vi "DetermineRegime.vi"(4 "Input Data":T1, 6 "Debug with explicit inputs? (F)":bool, 8 "Last Commanded Boat Regime":T5={"Sailing Regime"=enum."Upwind - Starboard Tack", "Emergency Regimes"=enum."NO EMERGENCY", "Emergency?"=FALSE}, 10 "Desired Heading (deg)":dbl, 11 "NotifierReff":T2) -> (3 "Commanded Boat Regime":T5)   [LabVIEW 2013]
doc: "This VI takes in\n - Trusted absolute wind data (this may be from the wind sensor, or may be frozen from before if the sensor data is bad in a certain area)\n - Robot heading (compass, 0-360)\n - Desired heading (same 0-360)\n - Last commanded regime\n\nThis VI commands a regime, either steady-state or transistion, and tells the Sail and Rudder controller to execute that regime. Documented here: https://docs.google.com/file/d/0B6St7IDGiYunU3FLWTZHTUFHWHc/edit\n\nFeb. 2014, Eric Schneider"
uses:
  Data/TypeDefs/Boat Regimes.ctl
  Data/TypeDefs/Sailing Regimes.ctl
  Data/TypeDefs/Emergency Regimes.ctl
  Data/TypeDefs/Regime Boundaries.ctl
  Data/TypeDefs/Notifiers.ctl
  Data/TypeDefs/UTM Location.ctl
  Data/TypeDefs/Sail Set Suggestions.ctl
  Data/TypeDefs/Rudder Set Suggestions.ctl
  Data/TypeDefs/OverrideInformation.ctl
  Data/TypeDefs/OverrideMode.ctl
  Data/TypeDefs/MotorSetup.ctl
  Data/TypeDefs/DynamixelSetupInfo.ctl
  Data/TypeDefs/AirmarStatus.ctl
panel:
  in  "Allowable Turn Error":dbl=5.0
  out "HasTransitionFailed?":bool
  out "Altered regime boundaries":T3=[0, 70, 140, 220, 190, 360]
  out "ShouldWeChangeRegime?":bool
  out "Desired Steady State Regime":T4
  out "Current Steady-State Regime":T4
  out "Are We In Transition?":bool
  # "These controls are only used for debugging, see the Midbrain Tests folder"
  # "FOR DEBUGGING"
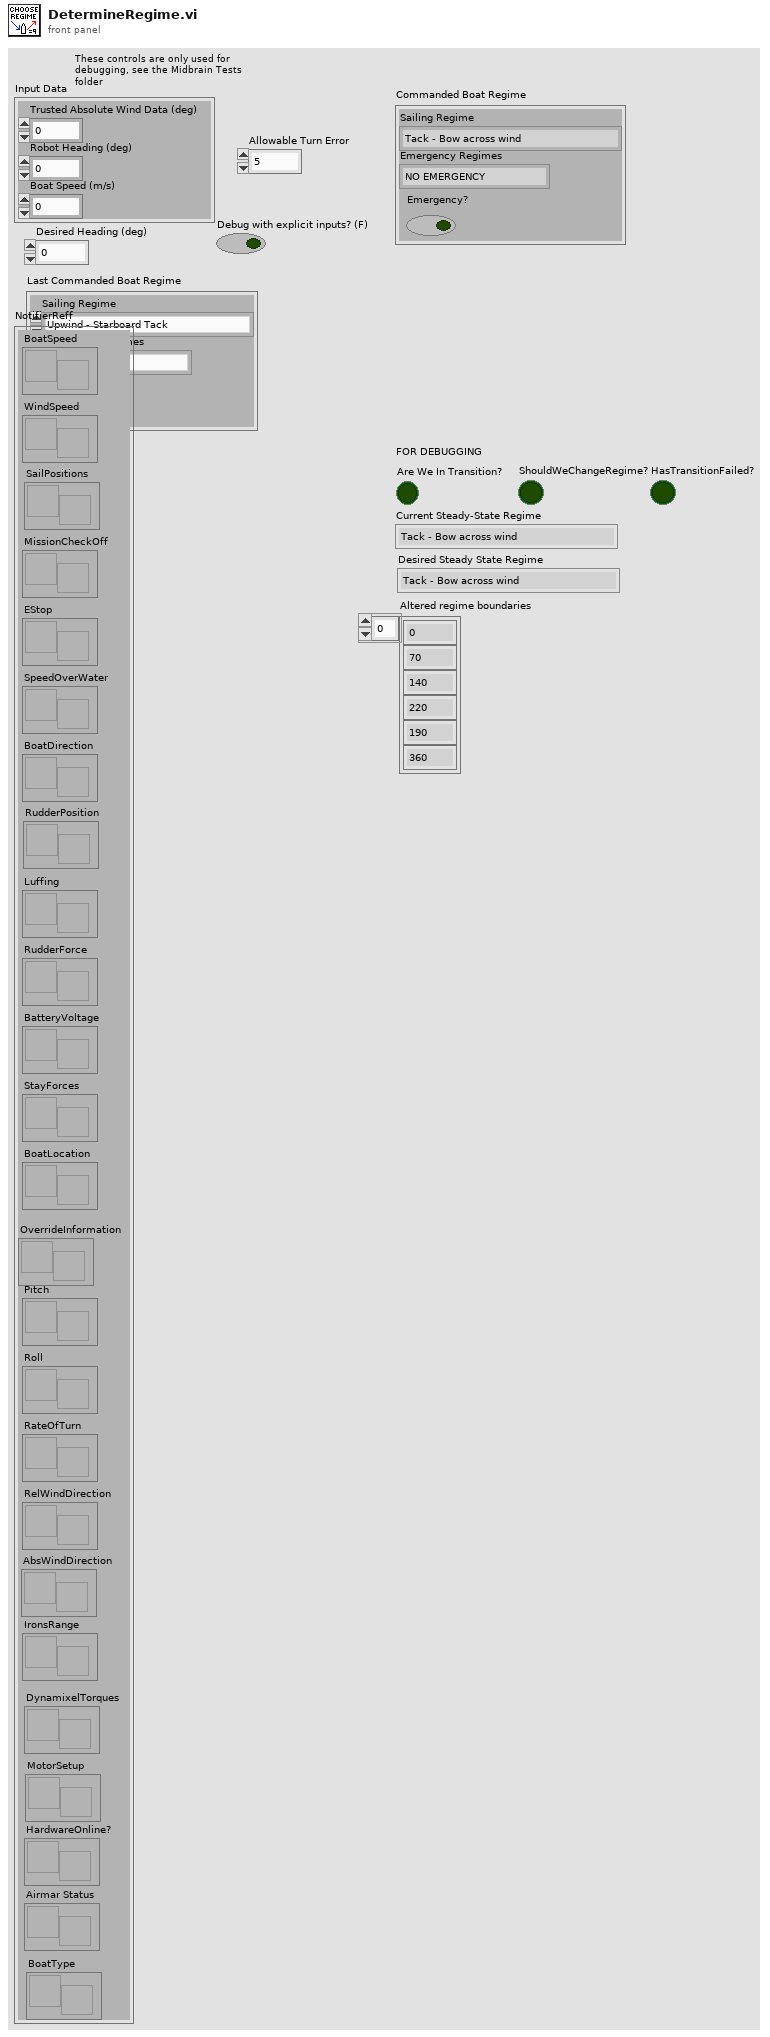
[diagram p1: front panel]
types:
  T1 = cluster{"Trusted Absolute Wind Data (deg)":dbl, "Robot Heading (deg)":dbl, "Boat Speed (m/s)":dbl}
  T2 = typedef "Notifiers.ctl" = cluster{"BoatSpeed":refnum<notifier>, "WindSpeed":refnum<notifier>, "MissionCheckOff":refnum<notifier>, "EStop":refnum<notifier>, "SpeedOverWater":refnum<notifier>, "BoatDirection":refnum<notifier>, "Luffing":refnum<notifier>, "RudderForce":refnum<notifier>, "BatteryVoltage":refnum<notifier>, "StayForces":refnum<notifier>, "BoatLocation":refnum<notifier>, "Pitch":refnum<notifier>, "Roll":refnum<notifier>, "RateOfTurn":refnum<notifier>, "RelWindDirection":refnum<notifier>, "SailPositions":refnum<notifier>, "RudderPosition":refnum<notifier>, "IronsRange":refnum<notifier>, "AbsWindDirection":refnum<notifier>, "OverrideInformation":refnum<notifier>, "DynamixelTorques":refnum<notifier>, "HardwareOnline?":refnum<notifier>, "MotorSetup":refnum<notifier>, "Airmar Status":refnum<notifier>, "BoatType":refnum<notifier>}
  T3 = typedef "Regime Boundaries.ctl" = i32[]
  T4 = typedef "Sailing Regimes.ctl" = enum16{"Tack - Bow across wind", "Upwind - Starboard Tack", "Turn between Upwind/Reach - Starboard Tack", "Reach - Starboard Tack", "Turn between Reach/Run - Starboard Tack", "Run - Starboard Tack", "Jibe - Stern across wind", "Run - Port Tack", "Turn between Reach/Run - Port Tack", "Reach - Port Tack", "Turn between Upwind/Reach - Port Tack", "Upwind - Port Tack"}
  T5 = typedef "Boat Regimes.ctl" = cluster{"Sailing Regime":T4, "Emergency Regimes":T6, "Emergency?":bool}
  T6 = typedef "Emergency Regimes.ctl" = enum16{"NO EMERGENCY", "No Knockdown", "Obstacle Avoid"}
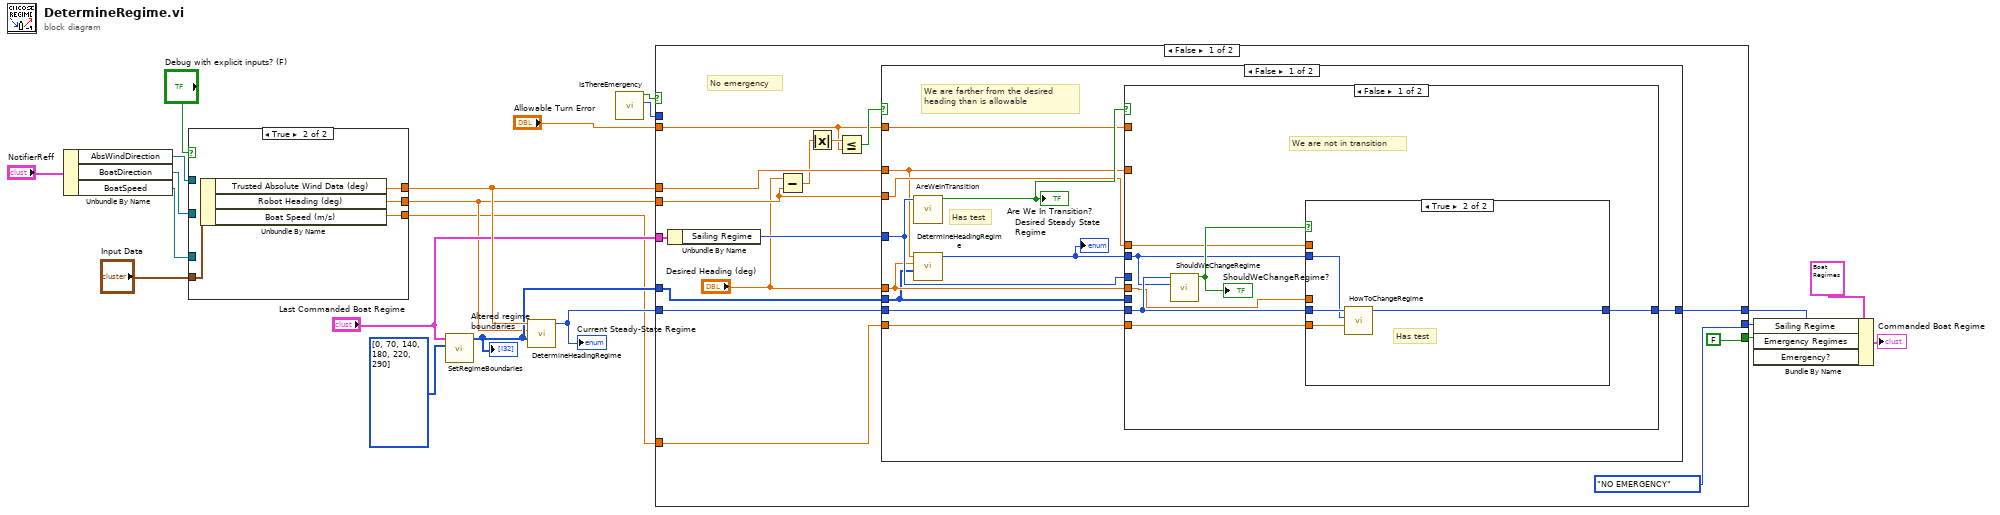
[diagram p0: block diagram]
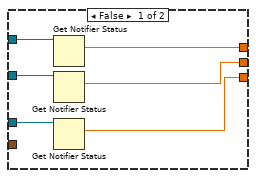
[diagram p2: hidden frame]
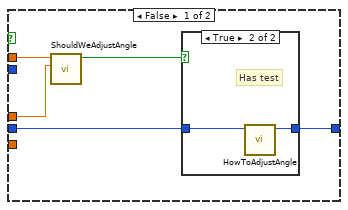
[diagram p3: hidden frame]
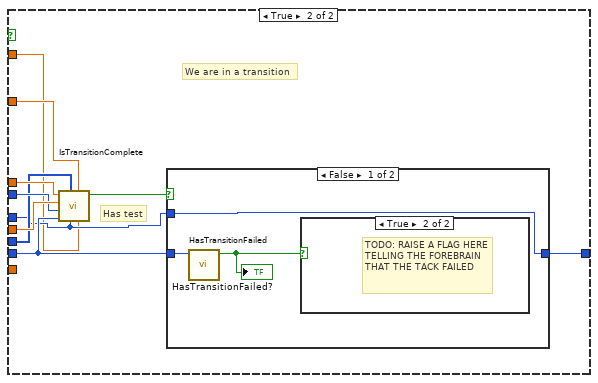
[diagram p5: hidden frame]
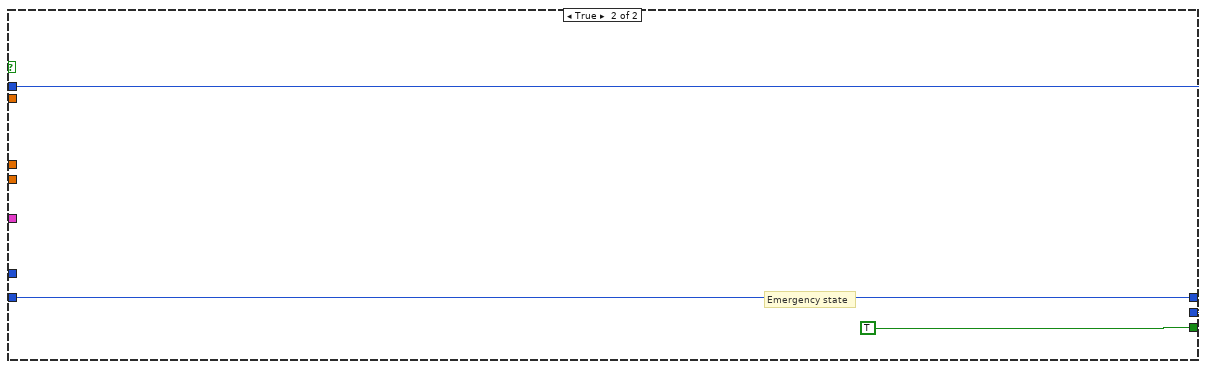
[diagram p9: hidden frame]
diagram:
  n1 = Unbundle By Name("NotifierReff") -> ("AbsWindDirection"=w5:refnum<notifier>, "BoatDirection"=w4:refnum<notifier>, "BoatSpeed"=w3:refnum<notifier>)
  n2 = case shown="True" "Debug with explicit inputs? (F)" {
    tunnel: [w27 w30] -> w13
    tunnel: [w26 w29] -> w8
    tunnel: w5 -> [w25 _]
    tunnel: w4 -> [w24 _]
    tunnel: w3 -> [w23 _]
    tunnel: [w22 w28] -> w2
    tunnel: "Input Data" -> [_ w31]
    frame False {
      n3 = Get Notifier Status(notifier=w25) -> (current notification=w27:dbl)  [unwired: 1 in, 4 out]
      n4 = Get Notifier Status(notifier=w24) -> (current notification=w26:dbl)  [unwired: 1 in, 4 out]
      n5 = Get Notifier Status(notifier=w23) -> (current notification=w22:dbl)  [unwired: 1 in, 4 out]
    }
    frame True {
      n6 = Unbundle By Name(w31) -> ("Trusted Absolute Wind Data (deg)"=w30:dbl, "Robot Heading (deg)"=w29:dbl, "Boat Speed (m/s)"=w28:dbl)
    }
  }
  n7 = call "SetRegimeBoundaries.vi"("Default regime boundaries"=T3 [0, 70, 140, 180, 220, 290], "Last Commanded Boat Regime"="Last Commanded Boat Regime") -> ("Altered regime boundaries"=w10:T3)  [unwired: 9 in]
  "Altered regime boundaries" <- w10
  n8 = call "DetermineHeadingRegime.vi"("Altered regime boundaries"=w10, "Robot Heading (deg)"=w8, "Trusted Absolute Wind Data (deg)"=w13) -> ("Sailing Regime"=w14:T4)  [unwired: 8 in]
  "Current Steady-State Regime" <- w14
  n9 = call "IsThereEmergency.vi"() -> ("Emergency Regime"=w15:T6, "Is There An Emergency?"=w21:bool)  [unwired: 10 in]
  n10 = case shown="False" w21 {
    tunnel: [w46 w92] -> w19
    tunnel: "Last Commanded Boat Regime" -> [w45 _]
    tunnel: [Emergency_Regimes."NO EMERGENCY" ("Emergency Regimes") w93] -> w16
    tunnel: [FALSE TRUE] -> w17
    tunnel: w15 -> [_ w93]
    tunnel: w14 -> [w41 w92]
    tunnel: w8 -> [w36 _]
    tunnel: w13 -> [w40 _]
    tunnel: w10 -> [w39 _]
    tunnel: "Allowable Turn Error" -> [w33 _]
    tunnel: w2 -> [w32 _]
    frame False {
      # "No emergency"
      n11 = Unbundle By Name(w45) -> ("Sailing Regime"=w44:T4)
      n12 = Subtract(x="Desired Heading (deg)", y=w36) -> (x-y=w38:dbl)
      n13 = Absolute Value(x=w38) -> (abs(x)=w34:dbl)
      n14 = Less Or Equal?(x=w34, y=w33) -> (x <= y?=w37:bool)
      n15 = case shown="False" w37 {
        tunnel: [w56 w91] -> w46
        tunnel: w44 -> [w55 _]
        tunnel: w41 -> [w54 w91]
        tunnel: w36 -> [w53 _]
        tunnel: w40 -> [w52 _]
        tunnel: "Desired Heading (deg)" -> [w51 _]
        tunnel: w39 -> [w50 _]
        tunnel: w33 -> [w48 _]
        tunnel: w32 -> [w47 _]
        frame False {
          # "We are farther from the desired heading than is allowable"
          # "Has test"
          n16 = call "AreWeInTransition.vi"("Last Commanded Sailing Regime"=w55) -> ("Are We In Transition?"=w57:bool)  [unwired: 10 in]
          "Are We In Transition?" <- w57
          n17 = call "DetermineHeadingRegime.vi"("Altered regime boundaries"=w50, "Robot Heading (deg)"=w51, "Trusted Absolute Wind Data (deg)"=w52) -> ("Sailing Regime"=w49:T4)  [unwired: 8 in]
          "Desired Steady State Regime" <- w49
          n18 = case shown="False" w57 {
            tunnel: w54 -> [w63 w81]
            tunnel: [w62 w86] -> w56
            tunnel: w51 -> [w60 w84]
            tunnel: w55 -> [_ w79]
            tunnel: w53 -> [w61 w83]
            tunnel: w52 -> [_ w78]
            tunnel: w49 -> [w59 w82]
            tunnel: w50 -> [_ w80]
            tunnel: w48 -> [_ w77]
            tunnel: w47 -> [w58 _]
            frame False {
              # "We are not in transition"
              n19 = call "ShouldWeChangeRegime.vi"("Desired Sailing Regime"=w59, "Current Sailing Regime"=w63) -> ("ShouldWeChangeRegime?"=w64:bool)  [unwired: 9 in]
              "ShouldWeChangeRegime?" <- w64
              n20 = case shown="True" w64 {
                tunnel: w63 -> [w67 w76]
                tunnel: w59 -> [_ w75]
                tunnel: [w66 w74] -> w62
                tunnel: w60 -> [w68 _]
                tunnel: w61 -> [w65 _]
                tunnel: w58 -> [_ w73]
                frame False {
                  n21 = call "ShouldWeAdjustAngle.vi"("DesiredHeading (0-360)"=w68, "RobotHeading (0-360)"=w65) -> ("ShouldWeAdjustAngle?"=w69:bool)  [unwired: 9 in]
                  n22 = case shown="True" w69 {
                    tunnel: w67 -> [w70 w72]
                    tunnel: [w70 w71] -> w66
                    frame False {
                    }
                    frame True {
                      # "Has test"
                      n23 = call "HowToAdjustAngle.vi"("Current Sailing Regime"=w72) -> ("Desired Sailing Regime"=w71:T4)  [unwired: 10 in]
                    }
                  }
                }
                frame True {
                  # "Has test"
                  n24 = call "HowToChangeRegime.vi"("Boat speed (m/s)"=w73, "Desired Sailing Regime"=w75, "Current Sailing Regime"=w76) -> ("Output sailing regime"=w74:T4)  [unwired: 8 in]
                }
              }
            }
            frame True {
              # "We are in a transition"
              # "Has test"
              n25 = call "IsTransitionComplete.vi"("Cutoff Range For Completion (deg)"=w77, "Trusted Absolute Wind (deg)"=w78, "Last Commanded Regime"=w79, "Altered regime boundaries"=w80, "Current Regime"=w81, "Desired Regime"=w82, "Desired Heading (deg)"=w84, "Robot Heading (deg)"=w83) -> ("Is Transition Complete?"=w85:bool)  [unwired: 3 in]
              n26 = case shown="False" w85 {
                tunnel: w81 -> [w89 w90]
                tunnel: [w88 w90] -> w86
                tunnel: w79 -> [w88 _]
                frame False {
                  n27 = call "HasTransitionFailed.vi"("Last Commanded Sailing Regime"=w89) -> ("HasTransitionFailed?"=w87:bool)  [unwired: 10 in]
                  "HasTransitionFailed?" <- w87
                  n28 = case shown="True" w87 {
                    frame False {
                    }
                    frame True {
                      # "TODO: RAISE A FLAG HERE TELLING THE FOREBRAIN THAT THE TACK FAILED"
                    }
                  }
                }
                frame True {
                }
              }
            }
          }
        }
        frame True {
          # "If the difference between the current and desired is negligible, stay in the same regime."
        }
      }
    }
    frame True {
      # "Emergency state"
    }
  }
  n29 = Bundle By Name(cluster=T5 {"Sailing Regime"=enum."Tack - Bow across wind", "Emergency Regimes"=enum."No Knockdown", "Emergency?"=FALSE} ("output cluster 2"), "Sailing Regime"=w19, "Emergency Regimes"=w16, "Emergency?"=w17) -> (→"Commanded Boat Regime":T5)
